vi "pid_manual_motion.vi"(8 "inputValid":bool=TRUE, 9 "lastPosValid":bool=TRUE, 10 "lastPos":fxp<+/-,32,4>, 11 "manualMotion":T1) -> (0 "moving":bool, 1 "outputValid":bool, 3 "output":fxp<+/-,32,4>)   [LabVIEW 2016]
uses:
  <vilib>/rvi/Memory/Memory_Emulation/nirvimemoryFastEmulation.vi
  <vilib>/rvi/Memory/Memory_Emulation/nirvimemoryEmulation.vi
  <vilib>/rvi/Emulation/niFpgaEmulationIsFPGAContextNoSignature.vi
  <vilib>/rvi/DataTransferAndStorage/Container/Common/niFpgaContainerGetUniqueNameForEmu.vi
  <vilib>/rvi/Emulation/niFpgaProcessEmulError.vi
  <vilib>/rvi/Emulation/niFpgaSctlEmulationGetInTimedLoop.vi
  <vilib>/rvi/errors/nirviReportUnexpectedCaseInternalError (U32).vi
  <vilib>/rvi/FXPMathLib/FxpSub/XNode/nifxpmath_Sub.xnode
  <vilib>/rvi/FXPMathLib/FxpMul/XNode/nifxpmath_Multiplier.xnode
  <vilib>/rvi/FXPMathLib/FxpAdd/XNode/nifxpmath_Add.xnode
  <vilib>/rvi/DataTransferAndStorage/Container/XNode/niFpgaContainer.xnode
  <instrlib>/_niInstr/Basic Elements/v1/FPGA/niInstr Basic Elements v1 FPGA.lvlib
  <vilib>/rvi/FXPMathLib/sim/FxpSim.dll
panel:
  out "index":u16
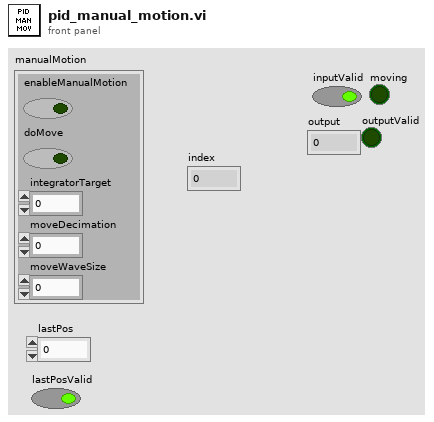
[diagram p1: front panel]
types:
  T1 = cluster{"enableManualMotion":bool, "doMove":bool, "integratorTarget":fxp<+/-,22,2>, "moveDecimation":u16, "moveWaveSize":u16}
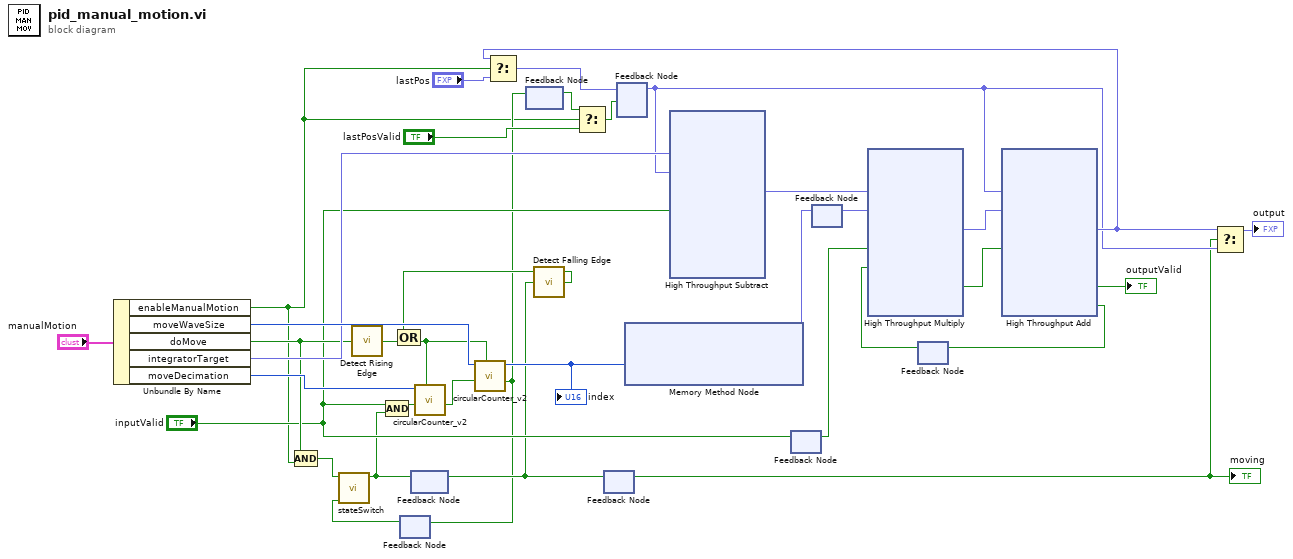
[diagram p0: block diagram]
diagram:
  n1 = Unbundle By Name("manualMotion") -> ("enableManualMotion"=w1:bool, "moveWaveSize"=w35:u16, "doMove"=w23:bool, "integratorTarget"=w34:fxp<+/-,22,2>, "moveDecimation"=w28:u16)
  n2 = Compound Arithmetic op=AND(w23, w1) -> (w2:bool)
  n3 = call <instrlib>:"Detect Rising Edge.vi"("signal"=w23) -> ("edge detected"=w22:bool)  [unwired: 14 in]
  n4 = feedback #1() -> (w24:bool)  [unwired: 1 in]
  n5 = call "stateSwitch.vi"("disable"=w24, "enable"=w2) -> ("state"=w7:bool)  [unwired: 9 in]
  n6 = Compound Arithmetic op=AND("inputValid", w7) -> (w8:bool)
  n7 = feedback #2() -> (w9:bool)  [unwired: 1 in]
  n8 = feedback-in #2(w7) -> ()
  n9 = feedback #3() -> (w3:bool)  [unwired: 1 in]
  n10 = call <instrlib>:"Detect Falling Edge.vi"("signal"=w9) -> ("edge detected"=w5:bool)  [unwired: 14 in]
  n11 = Compound Arithmetic op=OR(w5, w22) -> (w6:bool)
  n12 = call "circularCounter_v2.vi"("reset"=w6, "doStep"=w8, "maxCount"=w28) -> ("maxPulse"=w25:bool)  [unwired: 5 in, 3 out]
  n13 = call "circularCounter_v2.vi"("reset"=w6, "doStep"=w25, "maxCount"=w35) -> ("maxPulse"=w4:bool, "index"=w27:u16)  [unwired: 5 in, 2 out]
  "index" <- w27
  n14 = feedback-in #1(w4) -> ()
  n15 = feedback-in #3(w4) -> ()
  n16 = Select(t=w3, s=w1, f="lastPosValid") -> (s? t:f=w16:bool)
  n17 = feedback #4() -> (w10:bool)  [unwired: 1 in]
  "moving" <- w10
  n18 = feedback-in #4(w9) -> ()
  n19 = feedback #5() -> (w11:fxp<+/-,32,4>)  [unwired: 1 in]
  n20 = xnode ("Memory Method Node")("Address"=w27) -> ("Data"=w33:fxp<+/-,19,2>)  [unwired: 1 in, 1 out]
  n21 = xnode ("High Throughput Subtract")("x"=w34, "y"=w11, "input valid"="inputValid") -> ("x-y"=w32:fxp<+/-,22,2>)  [unwired: 1 in, 2 out]
  n22 = feedback #6() -> (w18:bool)  [unwired: 1 in]
  n23 = feedback-in #6("inputValid") -> ()
  n24 = feedback #7() -> (w21:fxp<+/-,19,2>)  [unwired: 1 in]
  n25 = feedback-in #7(w33) -> ()
  n26 = feedback #8() -> (w29:bool)  [unwired: 1 in]
  n27 = xnode ("High Throughput Multiply")("x"=w32, "y"=w21, "input valid"=w18, "ready for output (T)"=w29) -> ("x*y"=w26:fxp<+/-,22,2>, "output valid"=w31:bool)  [unwired: 1 out]
  n28 = xnode ("High Throughput Add")("x"=w11, "y"=w26, "input valid"=w31) -> ("x+y"=w13:fxp<+/-,32,4>, "output valid"=→"outputValid":bool, "ready for input"=w30:bool)  [unwired: 1 in]
  n29 = Select(t=w13, s=w1, f="lastPos") -> (s? t:f=w17:fxp<+/-,32,4>)
  n30 = feedback-in #5(w17, w16) -> ()
  n31 = feedback-in #8(w30) -> ()
  n32 = Select(t=w13, s=w10, f=w11) -> (s? t:f=→"output":fxp<+/-,32,4>)
